vi "NT Client.vi"(4 "Update Time":i32=100, 9 "Client Name":string="Dashboard") -> (0 "error out":errorcluster)   [LabVIEW 2025]
doc: "Place this VI in the Dashboard or other client applications. Provide the robot IP address so that it can know where to find the server.\n\nYou normally want the restart option to be true, but if you have your own restart strategy, you can disable it. Tracing is useful when debugging. Similarly, the disconnect timout may need to be raised if setting breakpoints. The user event ref will publish the client activities so that other elements of the dashboard are notified when packets are processed."
uses:
  <vilib>/Rock Robotics/Network Tables/NT Globals.vi
  ntcoreffi.dll
  FRC_NetworkTablesLV.dll
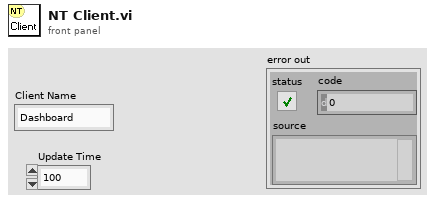
[diagram p1: front panel]
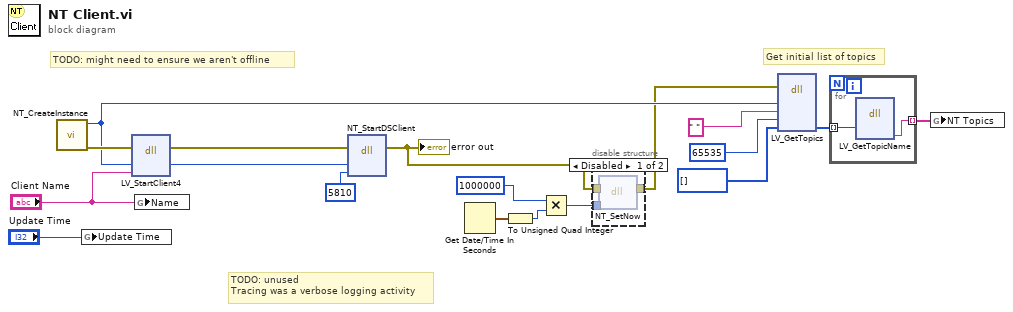
[diagram p0: block diagram]
diagram:
  # "Get initial list of topics"
  # "TODO: might need to ensure we aren't offline"
  # "TODO: unused\nTracing was a verbose logging activity"
  n1 = call <vilib>:"NT_CreateInstance.vi"() -> ("error out"=w17:errorcluster, "InstanceHandle"=w12:u64)  [unwired: 10 in]
  n2 = global write "NT Globals.vi" "Update Time"("Update Time") -> ()
  n3 = dll-call lib="FRC_NetworkTablesLV.*" fn="LV_StartClient4"(error in=w17, "InstHandle"=w12, "identity"="Client Name") -> (error out=w15:errorcluster, "InstHandle"=w16:u64)  [unwired: 4 in, 1 out]
  n4 = global write "NT Globals.vi" "Name"("Client Name") -> ()
  n5 = dll-call lib="ntcoreffi.*" fn="NT_StartDSClient"(error in=w15, "InstHandle"=w16, "port"=u32 5810) -> (error out=w2:errorcluster)  [unwired: 5 in, 1 out]
  "error out" <- w2
  n6 = Get Date/Time In Seconds() -> (seconds since 1Jan1904=w5:timestamp)
  n7 = To Unsigned Quad Integer(1:w5) -> (0:w6:u64)
  n8 = Multiply(x=u64 1000000, y=w6) -> (x*y=w3:u64)
  n9 = disable-structure shown="Disabled" {
    disable-tunnel: w3 -> [w21 _]
    disable-tunnel: w2 -> [w20 _]
    disable-tunnel: [w19 _] -> w1
    frame Disabled {
      n10 = dll-call lib="ntcoreffi.*" fn="NT_SetNow"(error in=w20, "fpgaTime"=w21) -> (error out=w19:errorcluster)  [unwired: 4 in, 1 out]
    }
    frame Enabled {
    }
  }
  n11 = dll-call lib="FRC_NetworkTablesLV.*" fn="LV_GetTopics"(error in=w1, "inst"=w12, "prefix"=" ", "typeMask"=u32 65535, "topicsArray"=u32[] []) -> ("topicsArray"=w9:u32[])  [unwired: 6 in, 2 out]
  n12 = for {
    tunnel: [w22] -> w10 mode=indexing
    tunnel: w9 -> [w23] mode=indexing
    n13 = dll-call lib="FRC_NetworkTablesLV.*" fn="LV_GetTopicName"("topic"=w23) -> ("name"=w22:string)  [unwired: 6 in, 2 out]
  }
  n14 = global write "NT Globals.vi" "NT Topics"(w10) -> ()
